vi "Configure Dialog.vi"(8 "error in (no error)":errorcluster, 11 "Configure FM Source [FM] Msg in":refnum<class "Configure FM Source [FM] Msg.lvclass">) -> (0 "error out":errorcluster, 2 "Ok?":bool, 3 "Configure FM Source [FM] Msg out":refnum<class "Configure FM Source [FM] Msg.lvclass">)   [LabVIEW 2014, in "CS++Fgen.lvlib" / "Configure FM Source [FM] Msg.lvclass"]
uses:
  Configure FM Source [FM] Msg.lvclass
  Configure FM Source [FM] Msg.lvclass/Configure FM Source [FM] Msg.ctl
panel:
  in  "source (Internal)":i32(ring) caption="Source" items=["Internal", "External"]
  in  "Channel Name (\"\")":string="CHANNEL1" caption="Channel Name"
  in  "OK Button":bool
  in  "Cancel Button":bool
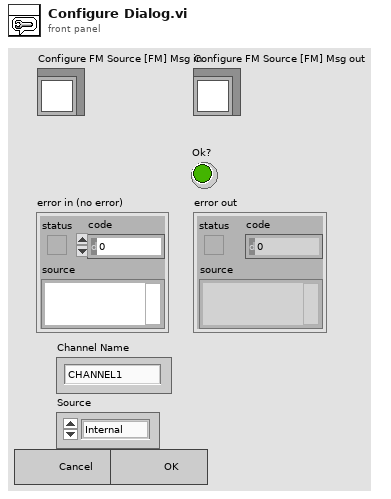
[diagram p1: front panel]
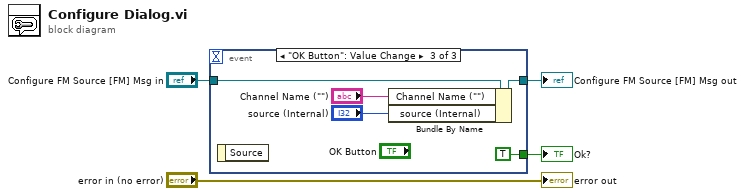
[diagram p0: block diagram]
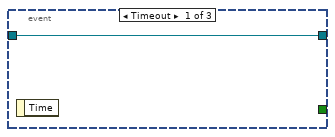
[diagram p2: hidden frame]
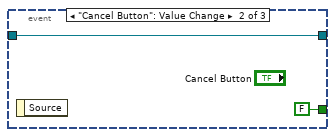
[diagram p3: hidden frame]
diagram:
  n1 = event shown="[2] \"OK Button\": Value Change" {
    selector: _ -> [_ _ _]
    dyn-events: _ -> [_ _ _]
    timeout: _ -> [_ _ _]
    tunnel: [w5 w7 w10] -> w3
    tunnel: "Configure FM Source [FM] Msg in" -> [w5 w7 w12]
    tunnel: [_ FALSE TRUE] -> w1
    event Timeout {
      n2 = event-data() -> ()  [unwired: 1 in, 1 out]
    }
    event "Cancel Button": Value Change {
      n3 = event-data() -> ()  [unwired: 1 in, 1 out]
    }
    event "OK Button": Value Change {
      n4 = event-data() -> ()  [unwired: 1 in, 1 out]
      n5 = Bundle By Name(cluster=w12, "Channel Name (\"\")"="Channel Name (\"\")", "source (Internal)"="source (Internal)") -> (w10:refnum<class "Configure FM Source [FM] Msg.lvclass">)
    }
  }
  "Configure FM Source [FM] Msg out" <- w3
  "Ok?" <- w1
  "error out" <- "error in (no error)"
